vi "API Tree.vi"   [LabVIEW 2019]
uses:
  src/Instrument.Lockin/Instrument.Lockin.lvclass
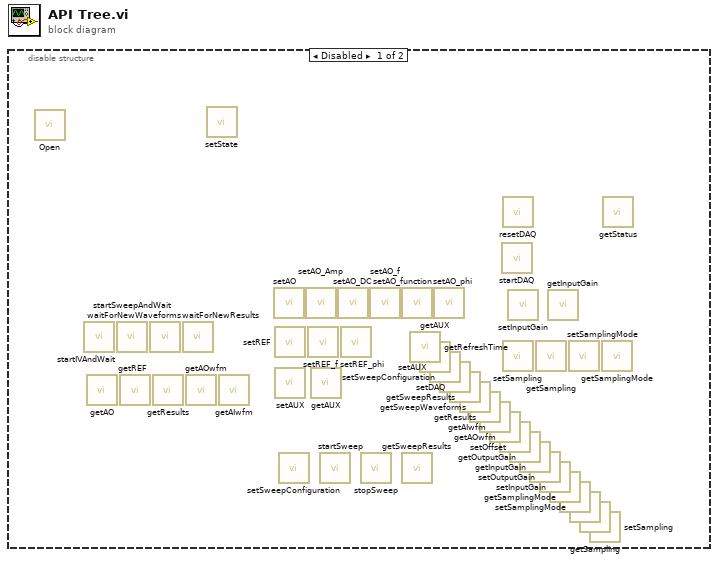
[diagram p0: block diagram]
diagram:
  n1 = disable-structure shown="Disabled" {
    frame Disabled {
      n2 = call-dynamic "Open.vi"() -> ()  [unwired: 10 in, 2 out]
      n3 = call "startIVAndWait.vi"() -> ()  [unwired: 9 in, 3 out]
      n4 = call "getAO.vi"() -> ()  [unwired: 9 in, 3 out]
      n5 = call "startSweepAndWait.vi"() -> ()  [unwired: 8 in, 4 out]
      n6 = call "getREF.vi"() -> ()  [unwired: 9 in, 3 out]
      n7 = call "waitForNewWaveforms.vi"() -> ()  [unwired: 9 in, 3 out]
      n8 = call "getResults.vi"() -> ()  [unwired: 8 in, 4 out]
      n9 = call "waitForNewResults.vi"() -> ()  [unwired: 9 in, 3 out]
      n10 = call "getAOwfm.vi"() -> ()  [unwired: 9 in, 3 out]
      n11 = call "setState.vi"() -> ()  [unwired: 10 in, 2 out]
      n12 = call "getAIwfm.vi"() -> ()  [unwired: 9 in, 3 out]
      n13 = call "setAO.vi"() -> ()  [unwired: 10 in, 2 out]
      n14 = call "setREF.vi"() -> ()  [unwired: 10 in, 2 out]
      n15 = call "setAUX.vi"() -> ()  [unwired: 10 in, 2 out]
      n16 = call "setSweepConfiguration.vi"() -> ()  [unwired: 10 in, 2 out]
      n17 = call "setAO_Amp.vi"() -> ()  [unwired: 10 in, 2 out]
      n18 = call "setREF_f.vi"() -> ()  [unwired: 10 in, 2 out]
      n19 = call "getAUX.vi"() -> ()  [unwired: 9 in, 3 out]
      n20 = call "startSweep.vi"() -> ()  [unwired: 10 in, 2 out]
      n21 = call "setAO_DC.vi"() -> ()  [unwired: 10 in, 2 out]
      n22 = call "setREF_phi.vi"() -> ()  [unwired: 10 in, 2 out]
      n23 = call "stopSweep.vi"() -> ()  [unwired: 10 in, 2 out]
      n24 = call "setAO_f.vi"() -> ()  [unwired: 10 in, 2 out]
      n25 = call "setAO_function.vi"() -> ()  [unwired: 10 in, 2 out]
      n26 = call "getSweepResults.vi"() -> ()  [unwired: 8 in, 4 out]
      n27 = call "getRefreshTime.vi"() -> ()  [unwired: 9 in, 3 out]
      n28 = call "getAUX.vi"() -> ()  [unwired: 9 in, 3 out]
      n29 = call "setAUX.vi"() -> ()  [unwired: 10 in, 2 out]
      n30 = call "setAO_phi.vi"() -> ()  [unwired: 10 in, 2 out]
      n31 = call "setSweepConfiguration.vi"() -> ()  [unwired: 10 in, 2 out]
      n32 = call "setDAQ.vi"() -> ()  [unwired: 10 in, 2 out]
      n33 = call "getSweepResults.vi"() -> ()  [unwired: 8 in, 4 out]
      n34 = call "getSweepWaveforms.vi"() -> ()  [unwired: 8 in, 4 out]
      n35 = call "getResults.vi"() -> ()  [unwired: 8 in, 4 out]
      n36 = call "getAIwfm.vi"() -> ()  [unwired: 9 in, 3 out]
      n37 = call "getAOwfm.vi"() -> ()  [unwired: 9 in, 3 out]
      n38 = call "startDAQ.vi"() -> ()  [unwired: 10 in, 2 out]
      n39 = call "resetDAQ.vi"() -> ()  [unwired: 10 in, 2 out]
      n40 = call "setSampling.vi"() -> ()  [unwired: 10 in, 2 out]
      n41 = call "setInputGain.vi"() -> ()  [unwired: 10 in, 2 out]
      n42 = call "setOffset.vi"() -> ()  [unwired: 10 in, 2 out]
      n43 = call "getOutputGain.vi"() -> ()  [unwired: 9 in, 3 out]
      n44 = call "getInputGain.vi"() -> ()  [unwired: 9 in, 3 out]
      n45 = call "getSampling.vi"() -> ()  [unwired: 9 in, 3 out]
      n46 = call "setOutputGain.vi"() -> ()  [unwired: 10 in, 2 out]
      n47 = call "getInputGain.vi"() -> ()  [unwired: 9 in, 3 out]
      n48 = call "setInputGain.vi"() -> ()  [unwired: 10 in, 2 out]
      n49 = call "getSamplingMode.vi"() -> ()  [unwired: 9 in, 3 out]
      n50 = call "setSamplingMode.vi"() -> ()  [unwired: 10 in, 2 out]
      n51 = call "setSamplingMode.vi"() -> ()  [unwired: 10 in, 2 out]
      n52 = call "getSampling.vi"() -> ()  [unwired: 9 in, 3 out]
      n53 = call "setSampling.vi"() -> ()  [unwired: 10 in, 2 out]
      n54 = call "getSamplingMode.vi"() -> ()  [unwired: 9 in, 3 out]
      n55 = call "getStatus.vi"() -> ()  [unwired: 9 in, 3 out]
    }
    frame Enabled {
    }
  }
